vi "Main-Get and Set Height-PD.vi"() -> ()   [LabVIEW 2014]
uses:
  Main-Stage-PI/(Global) Current handle and LaserPower_YCC.vi
  <vilib>/DAQmx/read.llb/DAQmx Read (Analog 2D DBL NChan NSamp).vi
  <vilib>/DAQmx/configure/trigger.llb/DAQmx Start Trigger (None).vi
panel:
  in  "Laser power":dbl
  out "inital Laser power":dbl
  out "Avg to Hz":dbl
  out "Expect - Real move (nm)\nStage Offset\n+=more move\n-=less move":dbl
  in  "Tab Control":enum32{"Raw QPDz-Stage", "Filtered QPDz-Stage"}(tab)
  out "Raw XY Graph":T1(graph)
  out "Filtered XY Graph":T1(graph)
  in  "Set Height":bool
  in  "Set Height (nm)":dbl=300.0
  in  "Avg points":i32=3000
  out "traveling time (s)":dbl
  in  "Sampling Rate":dbl=30000.0 format="%0.2f"
  out "Position after move up":dbl
  in  "1/2 range  (um)":dbl=0.8 format="%.3f"
  in  "scan rate  (um/s)":dbl=0.4 format="%.3f"
  out "Real Current Commanded position (um)":dbl format="%0.5f"
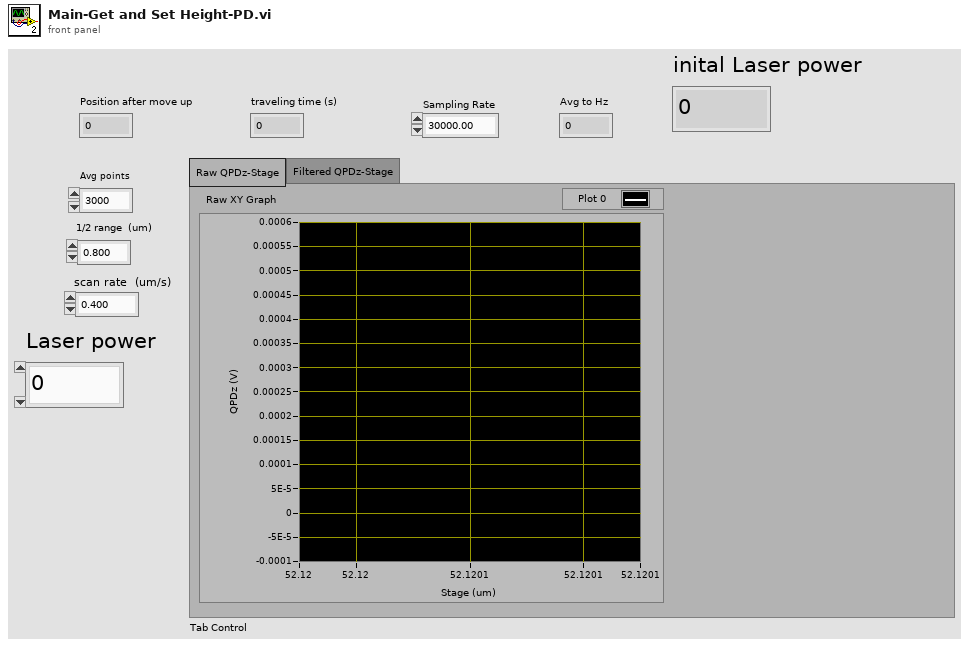
[diagram p1: front panel]
types:
  T1 = cluster{"Filtered Stage Array":dbl[], "Filtered QPD data":dbl[]}
  T2 = enum16{"Fixed-window avg", "Moving-window avg", "S-G filter", "Median filter"}
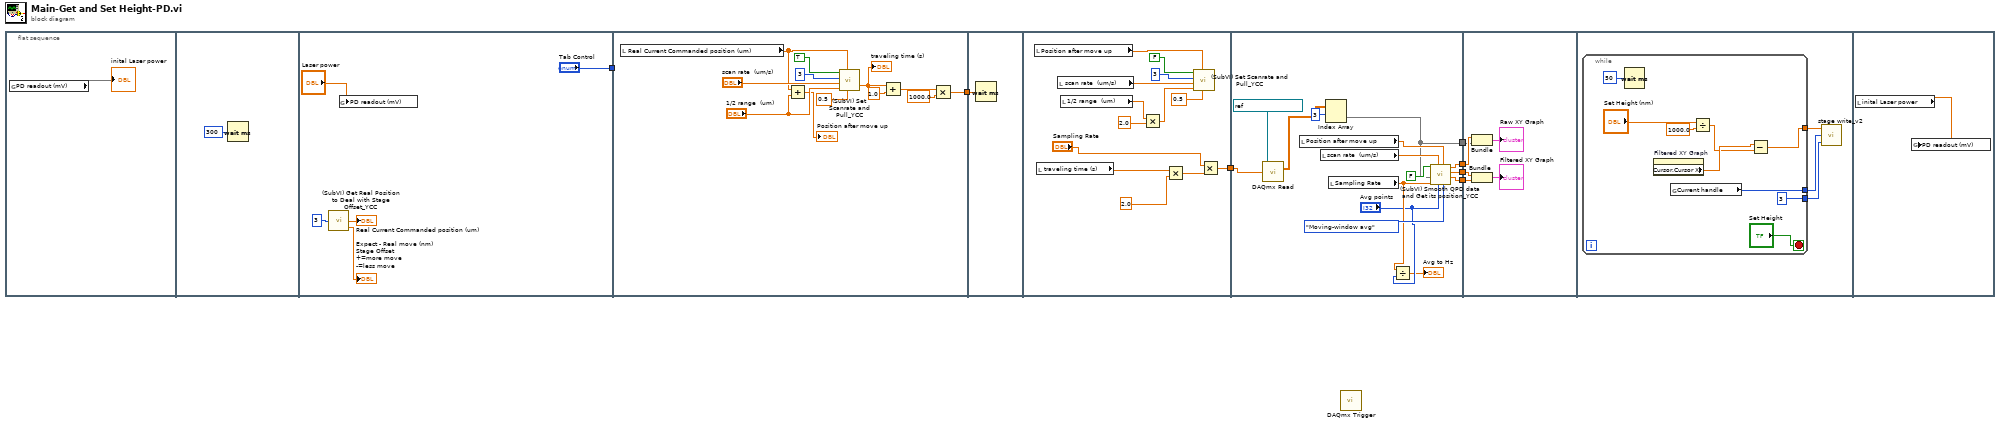
[diagram p0: block diagram]
diagram:
  n1 = flat-sequence {
    tunnel: ["Tab Control"] -> w1
    tunnel: [w19] -> w7
    tunnel: w1 -> [_]
    tunnel: w7 -> [w27]
    tunnel: [w36] -> w6
    tunnel: w6 -> [w55]
    tunnel: [w50] -> w5
    tunnel: [w49] -> w4
    tunnel: [w48] -> w3
    tunnel: [w41] -> w2
    tunnel: w5 -> [w61]
    tunnel: w4 -> [w60]
    tunnel: w3 -> [w59]
    tunnel: w2 -> [w58]
    frame #0 {
      n2 = global read "(Global) Current handle and LaserPower_YCC.vi" "PD readout (mV)"() -> (→"inital Laser power")
    }
    frame #1 {
      n3 = Wait (ms)(milliseconds to wait=u32 300) -> ()  [unwired: 1 out]
    }
    frame #2 {
      n4 = call "(SubVI) Get Real Position to Deal with Stage Offset_YCC.vi"("Axis"=3) -> ("Expect - Real move (nm)\nStage Offset\n+=more move\n-=less move"=→"Expect - Real move (nm)\nStage Offset\n+=more move\n-=less move":dbl, "Real Current Commanded position (um)"=→"Real Current Commanded position (um)":dbl)  [unwired: 3 in]
      n5 = global write "(Global) Current handle and LaserPower_YCC.vi" "PD readout (mV)"("Laser power") -> ()
    }
    frame #3 {
      n6 = local read "Real Current Commanded position (um)"() -> (w18:dbl)
      n7 = Add(x=w18, y="1/2 range  (um)") -> (x+y=→"Position after move up":dbl)
      n8 = call "(SubVI) Set Scanrate and Pull_YCC.vi"("waiting time per point (ms)\nrange from 5ms to 0.167 ms"=0.5 ("waiting time per point (ms)\nrange from 5ms to 0.167 ms"), "Start From  (um)"=w18, "range  (um)"="1/2 range  (um)", "scan rate  (um/s)"="scan rate  (um/s)", "axis"=u32 3, "toward+ ?\nT=+, F=-"=TRUE ("toward+ ?\nT=+, F=-")) -> ("traveling time (s)"=w15:dbl)  [unwired: 1 out]
      "traveling time (s)" <- w15
      n9 = Add(x=w15, y=1.0) -> (x+y=w21:dbl)
      n10 = Multiply(x=w21, y=1000.0) -> (x*y=w19:dbl)
    }
    frame #4 {
      n11 = Wait (ms)(milliseconds to wait=w27) -> ()  [unwired: 1 out]
    }
    frame #5 {
      n12 = local read "Position after move up"() -> (w35:dbl)
      n13 = local read "traveling time (s)"() -> (w30:dbl)
      n14 = local read "scan rate  (um/s)"() -> (w38:dbl)
      n15 = local read "1/2 range  (um)"() -> (w34:dbl)
      n16 = Multiply(x=w34, y=2.0) -> (x*y=w32:dbl)
      n17 = Multiply(x=w30, y=2.0) -> (x*y=w29:dbl)
      n18 = call "(SubVI) Set Scanrate and Pull_YCC.vi"("waiting time per point (ms)\nrange from 5ms to 0.167 ms"=0.5 ("waiting time per point (ms)\nrange from 5ms to 0.167 ms"), "Start From  (um)"=w35, "range  (um)"=w32, "scan rate  (um/s)"=w38, "axis"=u32 3, "toward+ ?\nT=+, F=-"=FALSE ("toward+ ?\nT=+, F=-")) -> ()  [unwired: 2 out]
      n19 = Multiply(x="Sampling Rate", y=w29) -> (x*y=w36:dbl)
    }
    frame #6 {
      n20 = call-poly <vilib>:"DAQmx Read.vi"("task/channels in"=refnum<k21> "PD-read-Task", "number of samples per channel"=w55) -> ("data"=w43:dbl[][])  [unwired: 11 in, 2 out]
      n21 = local read "Position after move up"() -> (w54:dbl)
      n22 = local read "scan rate  (um/s)"() -> (w53:dbl)
      n23 = Index Array(array=w43, index (row)=3) -> (element=w41:dbl[])  [unwired: 1 in]
      n24 = local read "Sampling Rate"() -> (w47:dbl)
      n25 = Divide(x=w47, y="Avg points") -> (x/y=→"Avg to Hz":dbl)
      n26 = call "(SubVI) Smooth QPD data and Get its position_YCC.vi"("Filter type"=T2."Moving-window avg", "Initial position (um)"=w54, "Avg points"="Avg points", "scan rate  (um/s)"=w53, "Sampling rate (Hz)"=w47, "QPD data"=w41, "Direction\nT=+ \nF=-"=FALSE ("T=+ first\nF=- first")) -> ("Filtered QPD data"=w49:dbl[], "Filtered Stage Array"=w50:dbl[], "Raw Stage Array"=w48:dbl[])  [unwired: 2 in]
    }
    frame #7 {
      n27 = Bundle("Raw Stage Array"=w59, "data"=w58) -> (→"Raw XY Graph":cluster{"Raw Stage Array":dbl[], "data":dbl[]})  [unwired: 1 in]
      n28 = Bundle("Filtered Stage Array"=w61, "Filtered QPD data"=w60) -> (→"Filtered XY Graph":T1)  [unwired: 1 in]
    }
    frame #8 {
      n29 = while {
        tunnel: [w73] -> w64
        tunnel: [w65] -> w63
        tunnel: [u32 3 ("axis")] -> w62
        stop <- "Set Height" stop-if-true
        n30 = Wait (ms)(milliseconds to wait=u32 50) -> ()  [unwired: 1 out]
        n31 = property on="Filtered XY Graph" class="XYGraph (strict)"() -> ("Cursor.Cursor X"=w67:dbl)  [unwired: 2 in, 2 out]
        n32 = global read "(Global) Current handle and LaserPower_YCC.vi" "Current handle"() -> (w73:i32)
        n33 = Divide(x="Set Height (nm)", y=1000.0) -> (x/y=w66:dbl)
        n34 = Subtract(x=w67, y=w66) -> (x-y=w65:dbl)
      }
      n35 = call "stage write_v2.vi"("axis"=w62, "Incoming Handle"=w64, "position"=w63) -> ()  [unwired: 2 in, 1 out]
    }
    frame #9 {
      n36 = local read "inital Laser power"() -> (w74:dbl)
      n37 = global write "(Global) Current handle and LaserPower_YCC.vi" "PD readout (mV)"(w74) -> ()
    }
  }
  n38 = call-poly <vilib>:"DAQmx Trigger.vi"() -> ()  [unwired: 14 in, 2 out]
